vi "Thread.Create.vi"(8 "error in (no error)":errorcluster, 9 "Processor (-2)":i32=-2, 10 "Priority (100)":i32=100, 11 "Thread type":refnum<class "Thread.lvclass">) -> (0 "error out":errorcluster, 3 "Thread":refnum<class "Thread.lvclass">)   [LabVIEW 2017, in "Thread.lvclass"]
uses:
  Thread.lvclass
  Thread.lvclass/Thread.ctl
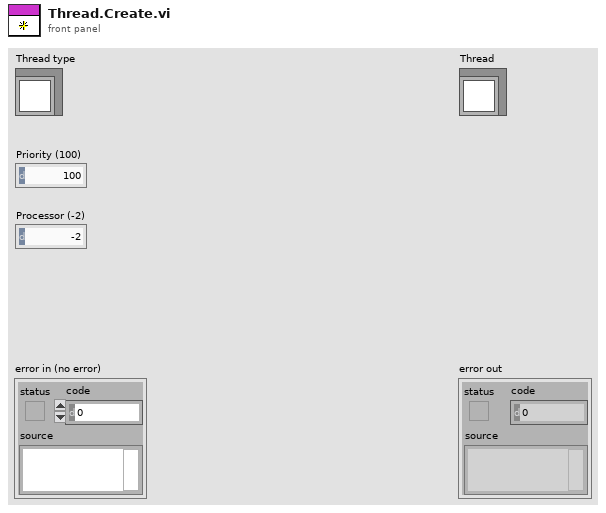
[diagram p1: front panel]
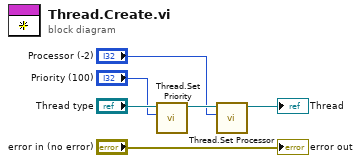
[diagram p0: block diagram]
diagram:
  n1 = call "Thread.Set Priority.vi"("Priority"="Priority (100)", "Thread in"="Thread type") -> ("Thread out"=w5:refnum<class "Thread.lvclass">)  [unwired: 9 in]
  n2 = call "Thread.Set Processor.vi"("Processor"="Processor (-2)", "Thread in"=w5) -> ("Thread out"=→"Thread":refnum<class "Thread.lvclass">)  [unwired: 9 in]
  "error out" <- "error in (no error)"
